vi "cRIO Input voltage.vi"(5 "DAQ_AI_Reader endpoint":refnum<k21>, 7 "Average":i32=1, 8 "error in (no error)":errorcluster, 11 "DAQ_CMD_Writer endpoint":refnum<k21>) -> (0 "error out":errorcluster, 2 "output cluster":T1, 3 "DAQ_CMD_Writer endpoint out":refnum<k21>)   [LabVIEW 2024]
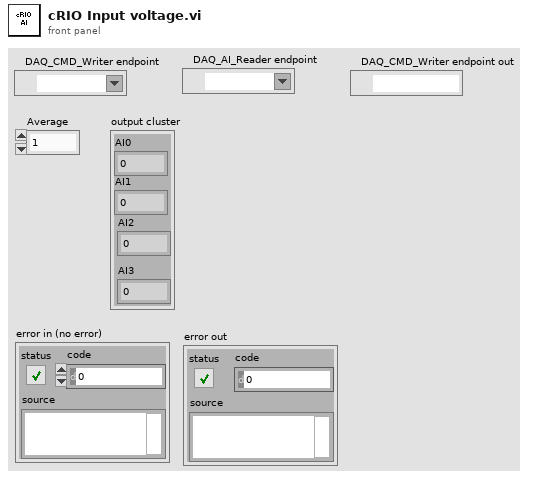
[diagram p1: front panel]
types:
  T1 = cluster{"AI0":dbl, "AI1":dbl, "AI2":dbl, "AI3":dbl}
  T2 = cluster{"Command":string, "Voltage":dbl, "Channel":string}
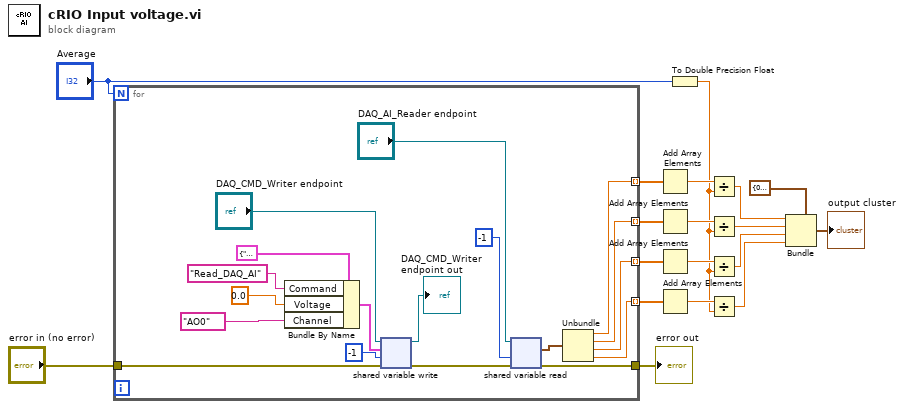
[diagram p0: block diagram]
diagram:
  n1 = for {
    N: "Average" -> [_]
    tunnel: "error in (no error)" -> [w34]
    tunnel: [w24] -> w17
    tunnel: [w22] -> w16 mode=indexing
    tunnel: [w21] -> w9 mode=indexing
    tunnel: [w20] -> w8 mode=indexing
    tunnel: [w19] -> w7 mode=indexing
    n2 = Bundle By Name(cluster=T2 {"Command"="", "Voltage"=0.0, "Channel"=""} ("output cluster"), "Command"="Read_DAQ_AI", "Voltage"=0.0, "Channel"="AO0" ("AO Channel")) -> (w28:T2)
    n3 = shared-variable-write("DAQ_CMD_Writer endpoint", w34, w28, -1 ("timeout ms (-1)")) -> (→"DAQ_CMD_Writer endpoint out":refnum<k21>, w25:errorcluster)  [unwired: 1 out]
    n4 = shared-variable-read("DAQ_AI_Reader endpoint", w25, -1 ("timeout ms (-1)")) -> (w24:errorcluster, w23:cluster{dbl, dbl, dbl, dbl})  [unwired: 2 out]
    n5 = Unbundle(w23) -> (w22:dbl, w21:dbl, w20:dbl, w19:dbl)
  }
  "error out" <- w17
  n6 = Add Array Elements(numeric array=w16) -> (sum=w15:dbl)
  n7 = Add Array Elements(numeric array=w9) -> (sum=w13:dbl)
  n8 = Add Array Elements(numeric array=w8) -> (sum=w12:dbl)
  n9 = Add Array Elements(numeric array=w7) -> (sum=w11:dbl)
  n10 = To Double Precision Float(number="Average") -> (double precision float=w10:dbl)
  n11 = Divide(x=w15, y=w10) -> (x/y=w5:dbl)
  n12 = Divide(x=w13, y=w10) -> (x/y=w4:dbl)
  n13 = Divide(x=w12, y=w10) -> (x/y=w3:dbl)
  n14 = Divide(x=w11, y=w10) -> (x/y=w2:dbl)
  n15 = Bundle(cluster=T1 {"AI0"=0.0, "AI1"=0.0, "AI2"=0.0, "AI3"=0.0} ("output cluster"), "AI0"=w5, "AI1"=w4, "AI2"=w3, "AI3"=w2) -> (→"output cluster":T1)
